vi "GeoData.vi"() -> ()   [LabVIEW 2017] (continued)
County\tH1\n26037\t54009\tFollansbee\tWV\tBrooke County\tH1\n26075\t54009\tWindsor heights\tWV\tBrooke County\tH1\n26062\t54009\tWeirton\tWV\tBrooke County\tH1\n26003\t54009\tWheeling\tWV\tBrooke County\tH1\n26030\t54009\tBeech bottom\tWV\tBrooke County\tH1\n26032\t54009\tBethany\tWV\tBrooke County\tH1\n26035\t54009\tColliers\tWV\tBrooke County\tH1\n26058\t54009\tShort creek\tWV\tBrooke County\tH1\n25504\t54011\tBarboursville\tWV\tCabell County\tH1\n25701\t54011\tHuntington\tWV\tCabell County\tH1\n25704\t54011\tHuntington\tWV\tCabell County\tH1\n26505\t54011\tMorgantown\tWV\tCabell County\tH1\n25723\t54011\tHuntington\tWV\tCabell County\tH1\n25711\t54011\tHuntington\tWV\tCabell County\tH1\n25727\t54011\tHuntington\tWV\tCabell County\tH1\n25702\t54011\tHuntington\tWV\tCabell County\tH1\n25703\t54011\tHuntington\tWV\tCabell County\tH1\n25713\t54011\tHuntington\tWV\tCabell County\tH1\n25779\t54011\tHuntington\tWV\tCabell County\tH1\n25772\t54011\tHuntington\tWV\tCabell County\tH1\n25716\t54011\tHuntington\tWV\tCabell County\tH1\n25715\t54011\tHuntington\tWV\tCabell County\tH1\n25526\t54011\tHurricane\tWV\tCabell County\tH1\n25510\t54011\tCulloden\tWV\tCabell County\tH1\n25714\t54011\tHuntington\tWV\tCabell County\tH1\n25778\t54011\tHuntington\tWV\tCabell County\tH1\n25728\t54011\tHuntington\tWV\tCabell County\tH1\n25755\t54011\tHuntington\tWV\tCabell County\tH1\n25706\t54011\tHuntington\tWV\tCabell County\tH1\n25719\t54011\tHuntington\tWV\tCabell County\tH1\n25729\t54011\tHuntington\tWV\tCabell County\tH1\n25775\t54011\tHuntington\tWV\tCabell County\tH1\n25545\t54011\tOna\tWV\tCabell County\tH1\n25708\t54011\tHuntington\tWV\tCabell County\tH1\n25721\t54011\tHuntington\tWV\tCabell County\tH1\n25726\t54011\tHuntington\tWV\tCabell County\tH1\n25725\t54011\tHuntington\tWV\tCabell County\tH1\n25717\t54011\tHuntington\tWV\tCabell County\tH1\n25773\t54011\tHuntington\tWV\tCabell County\tH1\n25541\t54011\tMilton\tWV\tCabell County\tH1\n25559\t54011\tSalt rock\tWV\tCabell County\tH1\n25520\t54011\tGlenwood\tWV\tCabell County\tH1\n25709\t54011\tHuntington\tWV\tCabell County\tH1\n25776\t54011\tHuntington\tWV\tCabell County\tH1\n25710\t54011\tHuntington\tWV\tCabell County\tH1\n25705\t54011\tHuntington\tWV\tCabell County\tH1\n25537\t54011\tLesage\tWV\tCabell County\tH1\n25777\t54011\tHuntington\tWV\tCabell County\tH1\n25707\t54011\tHuntington\tWV\tCabell County\tH1\n25712\t54011\tHuntington\tWV\tCabell County\tH1\n25722\t54011\tHuntington\tWV\tCabell County\tH1\n25506\t54011\tBranchland\tWV\tCabell County\tH1\n25718\t54011\tHuntington\tWV\tCabell County\tH1\n25720\t54011\tHuntington\tWV\tCabell County\tH1\n25724\t54011\tHuntington\tWV\tCabell County\tH1\n25774\t54011\tHuntington\tWV\tCabell County\tH1\n25235\t54013\tChloe\tWV\tCalhoun County\tH1\n25259\t54013\tLooneyville\tWV\tCalhoun County\tH1\n25261\t54013\tMillstone\tWV\tCalhoun County\tH1\n25141\t54013\tNebo\tWV\tCalhoun County\tH1\n26136\t54013\tBig bend\tWV\tCalhoun County\tH1\n25266\t54013\tNewton\tWV\tCalhoun County\tH1\n26147\t54013\tGrantsville\tWV\tCalhoun County\tH1\n26137\t54013\tBig springs\tWV\tCalhoun County\tH1\n26141\t54013\tCreston\tWV\tCalhoun County\tH1\n25234\t54013\tArnoldsburg\tWV\tCalhoun County\tH1\n26636\t54013\tRosedale\tWV\tCalhoun County\tH1\n26152\t54013\tMunday\tWV\tCalhoun County\tH1\n25276\t54013\tSpencer\tWV\tCalhoun County\tH1\n26151\t54013\tMount zion\tWV\tCalhoun County\tH1\n26138\t54013\tBrohard\tWV\tCalhoun County\tH1\n25268\t54013\tOrma\tWV\tCalhoun County\tH1\n25235\t54015\tChloe\tWV\tClay County\tH1\n25133\t54015\tMaysel\tWV\tClay County\tH1\n25125\t54015\tLizemores\tWV\tClay County\tH1\n25141\t54015\tNebo\tWV\tClay County\tH1\n25045\t54015\tClendenin\tWV\tClay County\tH1\n25043\t54015\tClay\tWV\tClay County\tH1\n25164\t54015\tProcious\tWV\tClay County\tH1\n25285\t54015\tWallback\tWV\tClay County\tH1\n25019\t54015\tBickmore\tWV\tClay County\tH1\n25088\t54015\tGlen\tWV\tClay County\tH1\n25113\t54015\tIvydale\tWV\tClay County\tH1\n25063\t54015\tDuck\tWV\tClay County\tH1\n26617\t54015\tDille\tWV\tClay County\tH1\n25111\t54015\tIndore\tWV\tClay County\tH1\n25030\t54015\tBomont\tWV\tClay County\tH1\n25211\t54015\tWiden\tWV\tClay County\tH1\n26321\t54017\tAlum bridge\tWV\tDoddridge County\tH1\n26443\t54017\tTroy\tWV\tDoddridge County\tH1\n26436\t54017\tSmithburg\tWV\tDoddridge County\tH1\n26415\t54017\tPennsboro\tWV\tDoddridge County\tH1\n26456\t54017\tWest union\tWV\tDoddridge County\tH1\n26411\t54017\tNew milton\tWV\tDoddridge County\tH1\n26426\t54017\tSalem\tWV\tDoddridge County\tH1\n26339\t54017\tCenter point\tWV\tDoddridge County\tH1\n26680\t54019\tNallen\tWV\tFayette County\tH1\n26656\t54019\tBelva\tWV\tFayette County\tH1\n25904\t54019\tPax\tWV\tFayette County\tH1\n25846\t54019\tGlen jean\tWV\tFayette County\tH1\n25002\t54019\tAlloy\tWV\tFayette County\tH1\n25031\t54019\tBoomer\tWV\tFayette County\tH1\n25801\t54019\tBeckley\tWV\tFayette County\tH1\n25840\t54019\tFayetteville\tWV\tFayette County\tH1\n25880\t54019\tMount hope\tWV\tFayette County\tH1\n26690\t54019\tSwiss\tWV\tFayette County\tH1\n25942\t54019\tWinona\tWV\tFayette County\tH1\n25936\t54019\tThurmond\tWV\tFayette County\tH1\n25901\t54019\tOak hill\tWV\tFayette County\tH1\n25119\t54019\tKincaid\tWV\tFayette County\tH1\n25186\t54019\tSmithers\tWV\tFayette County\tH1\n25831\t54019\tDanese\tWV\tFayette County\tH1\n25917\t54019\tScarbro\tWV\tFayette County\tH1\n25136\t54019\tMontgomery\tWV\tFayette County\tH1\n25083\t54019\tGallagher\tWV\tFayette County\tH1\n25115\t54019\tKanawha falls\tWV\tFayette County\tH1\n25938\t54019\tVictor\tWV\tFayette County\tH1\n25862\t54019\tLansing\tWV\tFayette County\tH1\n25139\t54019\tMount carbon\tWV\tFayette County\tH1\n25059\t54019\tDixie\tWV\tFayette County\tH1\n25866\t54019\tLochgelly\tWV\tFayette County\tH1\n25090\t54019\tGlen ferris\tWV\tFayette County\tH1\n25812\t54019\tAnsted\tWV\tFayette County\tH1\n25854\t54019\tHico\tWV\tFayette County\tH1\n25837\t54019\tEdmond\tWV\tFayette County\tH1\n25118\t54019\tKimberly\tWV\tFayette County\tH1\n25855\t54019\tHilltop\tWV\tFayette County\tH1\n25907\t54019\tPrince\tWV\tFayette County\tH1\n25879\t54019\tMinden\tWV\tFayette County\tH1\n25040\t54019\tCharlton heights\tWV\tFayette County\tH1\n25976\t54019\tMeadow bridge\tWV\tFayette County\tH1\n25161\t54019\tPowellton\tWV\tFayette County\tH1\n25173\t54019\tRobson\tWV\tFayette County\tH1\n25085\t54019\tGauley bridge\tWV\tFayette County\tH1\n25036\t54019\tCannelton\tWV\tFayette County\tH1\n25962\t54019\tRainelle\tWV\tFayette County\tH1\n25868\t54019\tLookout\tWV\tFayette County\tH1\n25185\t54019\tMount olive\tWV\tFayette County\tH1\n25888\t54019\tMount hope\tWV\tFayette County\tH1\n26412\t54021\tOrlando\tWV\tGilmer County\tH1\n26342\t54021\tCoxs mills\tWV\tGilmer County\tH1\n26384\t54021\tLinn\tWV\tGilmer County\tH1\n26443\t54021\tTroy\tWV\tGilmer County\tH1\n26638\t54021\tShock\tWV\tGilmer County\tH1\n26147\t54021\tGrantsville\tWV\tGilmer County\tH1\n26137\t54021\tBig springs\tWV\tGilmer County\tH1\n26335\t54021\tBurnsville\tWV\tGilmer County\tH1\n26430\t54021\tSand fork\tWV\tGilmer County\tH1\n26624\t54021\tGassaway\tWV\tGilmer County\tH1\n26611\t54021\tCedarville\tWV\tGilmer County\tH1\n26636\t54021\tRosedale\tWV\tGilmer County\tH1\n26351\t54021\tGlenville\tWV\tGilmer County\tH1\n26411\t54021\tNew milton\tWV\tGilmer County\tH1\n25267\t54021\tNormantown\tWV\tGilmer County\tH1\n26866\t54023\tUpper tract\tWV\tGrant County\tH1\n26717\t54023\tElk garden\tWV\tGrant County\tH1\n26855\t54023\tCabins\tWV\tGrant County\tH1\n26743\t54023\tNew creek\tWV\tGrant County\tH1\n26707\t54023\tBayard\tWV\tGrant County\tH1\n26739\t54023\tMount storm\tWV\tGrant County\tH1\n26720\t54023\tGormania\tWV\tGrant County\tH1\n26833\t54023\tMaysville\tWV\tGrant County\tH1\n26847\t54023\tPetersburg\tWV\tGrant County\tH1\n26836\t54023\tMoorefield\tWV\tGrant County\tH1\n26731\t54023\tLahmansville\tWV\tGrant County\tH1\n26710\t54023\tBurlington\tWV\tGrant County\tH1\n24977\t54025\tSmoot\tWV\tGreenbrier County\tH1\n26680\t54025\tNallen\tWV\tGreenbrier County\tH1\n24938\t54025\tFrankford\tWV\tGreenbrier County\tH1\n24901\t54025\tLewisburg\tWV\tGreenbrier County\tH1\n24931\t54025\tCrawley\tWV\tGreenbrier County\tH1\n26261\t54025\tRichwood\tWV\tGreenbrier County\tH1\n25981\t54025\tQuinwood\tWV\tGreenbrier County\tH1\n25984\t54025\tRupert\tWV\tGreenbrier County\tH1\n24966\t54025\tRenick\tWV\tGreenbrier County\tH1\n24957\t54025\tMaxwelton\tWV\tGreenbrier County\tH1\n24954\t54025\tMarlinton\tWV\tGreenbrier County\tH1\n24925\t54025\tCaldwell\tWV\tGreenbrier County\tH1\n24970\t54025\tRonceverte\tWV\tGreenbrier County\tH1\n25958\t54025\tCharmco\tWV\tGreenbrier County\tH1\n24916\t54025\tAsbury\tWV\tGreenbrier County\tH1\n25976\t54025\tMeadow bridge\tWV\tGreenbrier County\tH1\n24910\t54025\tAlderson\tWV\tGreenbrier County\tH1\n24986\t54025\tWhite sulphur springs\tWV\tGreenbrier County\tH1\n25962\t54025\tRainelle\tWV\tGreenbrier County\tH1\n24991\t54025\tWilliamsburg\tWV\tGreenbrier County\tH1\n24943\t54025\tGrassy meadows\tWV\tGreenbrier County\tH1\n25972\t54025\tLeslie\tWV\tGreenbrier County\tH1\n25434\t54027\tPaw paw\tWV\tHampshire County\tH1\n25422\t54027\tGreat cacapon\tWV\tHampshire County\tH1\n26704\t54027\tAugusta\tWV\tHampshire County\tH1\n26755\t54027\tRio\tWV\tHampshire County\tH1\n26711\t54027\tCapon bridge\tWV\tHampshire County\tH1\n26761\t54027\tShanks\tWV\tHampshire County\tH1\n26852\t54027\tPurgitsville\tWV\tHampshire County\tH1\n25437\t54027\tPoints\tWV\tHampshire County\tH1\n25431\t54027\tLevels\tWV\tHampshire County\tH1\n26808\t54027\tHigh view\tWV\tHampshire County\tH1\n26722\t54027\tGreen spring\tWV\tHampshire County\tH1\n26763\t54027\tSpringfield\tWV\tHampshire County\tH1\n26823\t54027\tCapon springs\tWV\tHampshire County\tH1\n25444\t54027\tSlanesville\tWV\tHampshire County\tH1\n26865\t54027\tYellow spring\tWV\tHampshire County\tH1\n26817\t54027\tBloomery\tWV\tHampshire County\tH1\n26757\t54027\tRomney\tWV\tHampshire County\tH1\n26710\t54027\tBurlington\tWV\tHampshire County\tH1\n26714\t54027\tDelray\tWV\tHampshire County\tH1\n26047\t54029\tNew cumberland\tWV\tHancock County\tH1\n26062\t54029\tWeirton\tWV\tHancock County\tH1\n26050\t54029\tNewell\tWV\tHancock County\tH1\n26056\t54029\tNew manchester\tWV\tHancock County\tH1\n26034\t54029\tChester\tWV\tHancock County\tH1\n26838\t54031\tMilam\tWV\tHardy County\tH1\n26755\t54031\tRio\tWV\tHardy County\tH1\n26851\t54031\tWardensville\tWV\tHardy County\tH1\n26818\t54031\tFisher\tWV\tHardy County\tH1\n26852\t54031\tPurgitsville\tWV\tHardy County\tH1\n26810\t54031\tLost city\tWV\tHardy County\tH1\n26845\t54031\tOld fields\tWV\tHardy County\tH1\n26812\t54031\tMathias\tWV\tHardy County\tH1\n26801\t54031\tBaker\tWV\tHardy County\tH1\n26847\t54031\tPetersburg\tWV\tHardy County\tH1\n26836\t54031\tMoorefield\tWV\tHardy County\tH1\n26815\t54031\tSugar grove\tWV\tHardy County\tH1\n26323\t54033\tAnmoore\tWV\tHarrison County\tH1\n26301\t54033\tClarksburg\tWV\tHarrison County\tH1\n26330\t54033\tBridgeport\tWV\tHarrison County\tH1\n26385\t54033\tLost creek\tWV\tHarrison County\tH1\n26416\t54033\tPhilippi\tWV\tHarrison County\tH1\n26361\t54033\tGypsy\tWV\tHarrison County\tH1\n26378\t54033\tJane lew\tWV\tHarrison County\tH1\n26582\t54033\tMannington\tWV\tHarrison County\tH1\n26386\t54033\tLumberport\tWV\tHarrison County\tH1\n26451\t54033\tWest milford\tWV\tHarrison County\tH1\n26456\t54033\tWest union\tWV\tHarrison County\tH1\n26438\t54033\tSpelter\tWV\tHarrison County\tH1\n26591\t54033\tWorthington\tWV\tHarrison County\tH1\n26422\t54033\tReynoldsville\tWV\tHarrison County\tH1\n26554\t54033\tFairmont\tWV\tHarrison County\tH1\n26568\t54033\tEnterprise\tWV\tHarrison County\tH1\n26306\t54033\tClarksburg\tWV\tHarrison County\tH1\n26426\t54033\tSalem\tWV\tHarrison County\tH1\n26366\t54033\tHaywood\tWV\tHarrison County\tH1\n26369\t54033\tHepzibah\tWV\tHarrison County\tH1\n26463\t54033\tWyatt\tWV\tHarrison County\tH1\n26408\t54033\tMount clare\tWV\tHarrison County\tH1\n26431\t54033\tShinnston\tWV\tHarrison County\tH1\n26448\t54033\tWallace\tWV\tHarrison County\tH1\n26404\t54033\tMeadowbrook\tWV\tHarrison County\tH1\n25252\t54035\tLe roy\tWV\tJackson County\tH1\n26169\t54035\tRockport\tWV\tJackson County\tH1\n25271\t54035\tRipley\tWV\tJackson County\tH1\n26164\t54035\tRavenswood\tWV\tJackson County\tH1\n25275\t54035\tSandyville\tWV\tJackson County\tH1\n25264\t54035\tMount alto\tWV\tJackson County\tH1\n25262\t54035\tMillwood\tWV\tJackson County\tH1\n25244\t54035\tGay\tWV\tJackson County\tH1\n25243\t54035\tGandeeville\tWV\tJackson County\tH1\n26143\t54035\tElizabeth\tWV\tJackson County\tH1\n26160\t54035\tPalestine\tWV\tJackson County\tH1\n25245\t54035\tGiven\tWV\tJackson County\tH1\n25241\t54035\tEvans\tWV\tJackson County\tH1\n25248\t54035\tKenna\tWV\tJackson County\tH1\n25124\t54035\tLiberty\tWV\tJackson County\tH1\n26133\t54035\tBelleville\tWV\tJackson County\tH1\n25239\t54035\tCottageville\tWV\tJackson County\tH1\n25231\t54035\tAdvent\tWV\tJackson County\tH1\n25414\t54037\tCharles town\tWV\tJefferson County\tH1\n25425\t54037\tHarpers ferry\tWV\tJefferson County\tH1\n25446\t54037\tSummit point\tWV\tJefferson County\tH1\n25443\t54037\tShepherdstown\tWV\tJefferson County\tH1\n25441\t54037\tRippon\tWV\tJefferson County\tH1\n25404\t54037\tMartinsburg\tWV\tJefferson County\tH1\n25442\t54037\tShenandoah junction\tWV\tJefferson County\tH1\n25432\t54037\tMillville\tWV\tJefferson County\tH1\n25430\t54037\tKearneysville\tWV\tJefferson County\tH1\n25438\t54037\tRanson\tWV\tJefferson County\tH1\n25423\t54037\tHalltown\tWV\tJefferson County\tH1\n25071\t54039\tElkview\tWV\tKanawha County\tH1\n25301\t54039\tCharleston\tWV\tKanawha County\tH1\n25312\t54039\tCharleston\tWV\tKanawha County\tH1\n25311\t54039\tCharleston\tWV\tKanawha County\tH1\n25320\t54039\tCharleston\tWV\tKanawha County\tH1\n25324\t54039\tCharleston\tWV\tKanawha County\tH1\n25326\t54039\tCharleston\tWV\tKanawha County\tH1\n25334\t54039\tCharleston\tWV\tKanawha County\tH1\n25336\t54039\tCharleston\tWV\tKanawha County\tH1\n25102\t54039\tHandley\tWV\tKanawha County\tH1\n25201\t54039\tTad\tWV\tKanawha County\tH1\n25143\t54039\tNitro\tWV\tKanawha County\tH1\n25075\t54039\tEskdale\tWV\tKanawha County\tH1\n25213\t54039\tWinfield\tWV\tKanawha County\tH1\n25303\t54039\tSouth charleston\tWV\tKanawha County\tH1\n25339\t54039\tCharleston\tWV\tKanawha County\tH1\n25321\t54039\tCharleston\tWV\tKanawha County\tH1\n25112\t54039\tInstitute\tWV\tKanawha County\tH1\n25327\t54039\tCharleston\tWV\tKanawha County\tH1\n25322\t54039\tCharleston\tWV\tKanawha County\tH1\n25328\t54039\tCharleston\tWV\tKanawha County\tH1\n25126\t54039\tLondon\tWV\tKanawha County\tH1\n25314\t54039\tCharleston\tWV\tKanawha County\tH1\n25306\t54039\tCharleston\tWV\tKanawha County\tH1\n25039\t54039\tCedar grove\tWV\tKanawha County\tH1\n25364\t54039\tCharleston\tWV\tKanawha County\tH1\n25361\t54039\tCharleston\tWV\tKanawha County\tH1\n25323\t54039\tCharleston\tWV\tKanawha County\tH1\n25335\t54039\tCharleston\tWV\tKanawha County\tH1\n25338\t54039\tCharleston\tWV\tKanawha County\tH1\n25045\t54039\tClendenin\tWV\tKanawha County\tH1\n25202\t54039\tTornado\tWV\tKanawha County\tH1\n25309\t54039\tSouth charleston\tWV\tKanawha County\tH1\n25286\t54039\tWalton\tWV\tKanawha County\tH1\n25387\t54039\tCharleston\tWV\tKanawha County\tH1\n25162\t54039\tPratt\tWV\tKanawha County\tH1\n25333\t54039\tCharleston\tWV\tKanawha County\tH1\n25362\t54039\tCharleston\tWV\tKanawha County\tH1\n25136\t54039\tMontgomery\tWV\tKanawha County\tH1\n25110\t54039\tHugheston\tWV\tKanawha County\tH1\n25083\t54039\tGallagher\tWV\tKanawha County\tH1\n25054\t54039\tDawes\tWV\tKanawha County\tH1\n25331\t54039\tCharleston\tWV\tKanawha County\tH1\n25159\t54039\tPoca\tWV\tKanawha County\tH1\n25305\t54039\tCharleston\tWV\tKanawha County\tH1\n25313\t54039\tCharleston\tWV\tKanawha County\tH1\n25330\t54039\tCharleston\tWV\tKanawha County\tH1\n25332\t54039\tCharleston\tWV\tKanawha County\tH1\n25325\t54039\tCharleston\tWV\tKanawha County\tH1\n25026\t54039\tBlue creek\tWV\tKanawha County\tH1\n25302\t54039\tCharleston\tWV\tKanawha County\tH1\n25025\t54039\tBlount\tWV\tKanawha County\tH1\n25160\t54039\tPond gap\tWV\tKanawha County\tH1\n25337\t54039\tCharleston\tWV\tKanawha County\tH1\n25317\t54039\tCharleston\tWV\tKanawha County\tH1\n25064\t54039\tDunbar\tWV\tKanawha County\tH1\n25177\t54039\tSaint albans\tWV\tKanawha County\tH1\n25248\t54039\tKenna\tWV\tKanawha County\tH1\n25124\t54039\tLiberty\tWV\tKanawha County\tH1\n25304\t54039\tCharleston\tWV\tKanawha County\tH1\n25107\t54039\tHernshaw\tWV\tKanawha County\tH1\n25389\t54039\tCharleston\tWV\tKanawha County\tH1\n25035\t54039\tCabin creek\tWV\tKanawha County\tH1\n25067\t54039\tEast bank\tWV\tKanawha County\tH1\n25061\t54039\tDrybranch\tWV\tKanawha County\tH1\n25015\t54039\tBelle\tWV\tKanawha County\tH1\n25003\t54039\tAlum creek\tWV\tKanawha County\tH1\n25214\t54039\tWinifrede\tWV\tKanawha County\tH1\n25315\t54039\tCharleston\tWV\tKanawha County\tH1\n25030\t54039\tBomont\tWV\tKanawha County\tH1\n25132\t54039\tMammoth\tWV\tKanawha County\tH1\n25103\t54039\tHansford\tWV\tKanawha County\tH1\n25329\t54039\tCharleston\tWV\tKanawha County\tH1\n25156\t54039\tPinch\tWV\tKanawha County\tH1\n25079\t54039\tFalling rock\tWV\tKanawha County\tH1\n25086\t54039\tGlasgow\tWV\tKanawha County\tH1\n25134\t54039\tMiami\tWV\tKanawha County\tH1\n25396\t54039\tCharleston\tWV\tKanawha County\tH1\n26321\t54041\tAlum bridge\tWV\tLewis County\tH1\n26412\t54041\tOrlando\tWV\tLewis County\tH1\n26384\t54041\tLinn\tWV\tLewis County\tH1\n26218\t54041\tFrench creek\tWV\tLewis County\tH1\n26372\t54041\tHorner\tWV\tLewis County\tH1\n26376\t54041\tIreland\tWV\tLewis County\tH1\n26378\t54041\tJane lew\tWV\tLewis County\tH1\n26452\t54041\tWeston\tWV\tLewis County\tH1\n26338\t54041\tCamden\tWV\tLewis County\tH1\n26447\t54041\tWalkersville\tWV\tLewis County\tH1\n26201\t54041\tBuckhannon\tWV\tLewis County\tH1\n26343\t54041\tCrawford\tWV\tLewis County\tH1\n26411\t54041\tNew milton\tWV\tLewis County\tH1\n25523\t54043\tHamlin\tWV\tLincoln County\tH1\n25529\t54043\tJulian\tWV\tLincoln County\tH1\n25521\t54043\tGriffithsville\tWV\tLincoln County\tH1\n25564\t54043\tSod\tWV\tLincoln County\tH1\n25526\t54043\tHurricane\tWV\tLincoln County\tH1\n25510\t54043\tCulloden\tWV\tLincoln County\tH1\n25573\t54043\tYawkey\tWV\tLincoln County\tH1\n25699\t54043\tWilsondale\tWV\tLincoln County\tH1\n25202\t54043\tTornado\tWV\tLincoln County\tH1\n25501\t54043\tAlkol\tWV\tLincoln County\tH1\n25524\t54043\tHarts\tWV\tLincoln County\tH1\n25313\t54043\tCharleston\tWV\tLincoln County\tH1\n25565\t54043\tSpurlockville\tWV\tLincoln County\tH1\n25567\t54043\tSumerco\tWV\tLincoln County\tH1\n25534\t54043\tKiahsville\tWV\tLincoln County\tH1\n25557\t54043\tRanger\tWV\tLincoln County\tH1\n25571\t54043\tWest hamlin\tWV\tLincoln County\tH1\n25540\t54043\tMidkiff\tWV\tLincoln County\tH1\n25544\t54043\tMyra\tWV\tLincoln County\tH1\n25003\t54043\tAlum creek\tWV\tLincoln County\tH1\n25506\t54043\tBranchland\tWV\tLincoln County\tH1\n25617\t54045\tDavin\tWV\tLogan County\tH1\n25634\t54045\tMallory\tWV\tLogan County\tH1\n25625\t54045\tHolden\tWV\tLogan County\tH1\n25505\t54045\tBig creek\tWV\tLogan County\tH1\n25612\t54045\tChauncey\tWV\tLogan County\tH1\n25653\t54045\tWilkinson\tWV\tLogan County\tH1\n25508\t54045\tChapmanville\tWV\tLogan County\tH1\n25547\t54045\tPecks mill\tWV\tLogan County\tH1\n25644\t54045\tSarah ann\tWV\tLogan County\tH1\n25022\t54045\tBlair\tWV\tLogan County\tH1\n25628\t54045\tKistler\tWV\tLogan County\tH1\n25524\t54045\tHarts\tWV\tLogan County\tH1\n25646\t54045\tStollings\tWV\tLogan County\tH1\n25047\t54045\tClothier\tWV\tLogan County\tH1\n25647\t54045\tSwitzer\tWV\tLogan County\tH1\n25639\t54045\tPeach creek\tWV\tLogan County\tH1\n25108\t54045\tHewett\tWV\tLogan County\tH1\n25652\t54045\tWhitman\tWV\tLogan County\tH1\n25606\t54045\tAccoville\tWV\tLogan County\tH1\n25614\t54045\tCora\tWV\tLogan County\tH1\n25649\t54045\tVerdunville\tWV\tLogan County\tH1\n25654\t54045\tYolyn\tWV\tLogan County\tH1\n25635\t54045\tMan\tWV\tLogan County\tH1\n25183\t54045\tSharples\tWV\tLogan County\tH1\n25607\t54045\tAmherstdale\tWV\tLogan County\tH1\n25601\t54045\tLogan\tWV\tLogan County\tH1\n25638\t54045\tOmar\tWV\tLogan County\tH1\n25121\t54045\tLake\tWV\tLogan County\tH1\n25670\t54045\tDelbarton\tWV\tLogan County\tH1\n25076\t54045\tEthel\tWV\tLogan County\tH1\n25632\t54045\tLyburn\tWV\tLogan County\tH1\n25637\t54045\tMount gay\tWV\tLogan County\tH1\n25611\t54045\tBruno\tWV\tLogan County\tH1\n25624\t54045\tHenlawson\tWV\tLogan County\tH1\n25630\t54045\tLorado\tWV\tLogan County\tH1\n24862\t54047\tMohawk\tWV\tMcDowell County\tH1\n24871\t54047\tPageton\tWV\tMcDowell County\tH1\n24831\t54047\tElkhorn\tWV\tMcDowell County\tH1\n24861\t54047\tMaybeury\tWV\tMcDowell County\tH1\n24881\t54047\tRoderfield\tWV\tMcDowell County\tH1\n24866\t54047\tNewhall\tWV\tMcDowell County\tH1\n24813\t54047\tBartley\tWV\tMcDowell County\tH1\n24811\t54047\tAvondale\tWV\tMcDowell County\tH1\n24817\t54047\tBradshaw\tWV\tMcDowell County\tH1\n24826\t54047\tCucumber\tWV\tMcDowell County\tH1\n24828\t54047\tDavy\tWV\tMcDowell County\tH1\n24879\t54047\tRaysal\tWV\tMcDowell County\tH1\n24846\t54047\tIsaban\tWV\tMcDowell County\tH1\n24855\t54047\tKyle\tWV\tMcDowell County\tH1\n24830\t54047\tElbert\tWV\tMcDowell County\tH1\n24829\t54047\tEckman\tWV\tMcDowell County\tH1\n24816\t54047\tBig sandy\tWV\tMcDowell County\tH1\n24873\t54047\tPaynesville\tWV\tMcDowell County\tH1\n24895\t54047\tWilcoe\tWV\tMcDowell County\tH1\n24878\t54047\tPremier\tWV\tMcDowell County\tH1\n24894\t54047\tWarriormine\tWV\tMcDowell County\tH1\n24808\t54047\tAnawalt\tWV\tMcDowell County\tH1\n24848\t54047\tJenkinjones\tWV\tMcDowell County\tH1\n24836\t54047\tGary\tWV\tMcDowell County\tH1\n24892\t54047\tWar\tWV\tMcDowell County\tH1\n24801\t54047\tWelch\tWV\tMcDowell County\tH1\n24872\t54047\tPanther\tWV\tMcDowell County\tH1\n24868\t54047\tNorthfork\tWV\tMcDowell County\tH1\n24815\t54047\tBerwind\tWV\tMcDowell County\tH1\n24850\t54047\tJolo\tWV\tMcDowell County\tH1\n24888\t54047\tThorpe\tWV\tMcDowell County\tH1\n24884\t54047\tSquire\tWV\tMcDowell County\tH1\n24844\t54047\tIaeger\tWV\tMcDowell County\tH1\n24853\t54047\tKimball\tWV\tMcDowell County\tH1\n24843\t54047\tHensley\tWV\tMcDowell County\tH1\n24887\t54047\tSwitchback\tWV\tMcDowell County\tH1\n26563\t54049\tCarolina\tWV\tMarion County\tH1\n26330\t54049\tBridgeport\tWV\tMarion County\tH1\n26508\t54049\tMorgantown\tWV\tMarion County\tH1\n26570\t54049\tFairview\tWV\tMarion County\tH1\n26588\t54049\tRivesville\tWV\tMarion County\tH1\n26562\t54049\tBurton\tWV\tMarion County\tH1\n26586\t54049\tMontana mines\tWV\tMarion County\tH1\n26559\t54049\tBarrackville\tWV\tMarion County\tH1\n26354\t54049\tGrafton\tWV\tMarion County\tH1\n26582\t54049\tMannington\tWV\tMarion County\tH1\n26576\t54049\tIdamay\tWV\tMarion County\tH1\n26572\t54049\tFour states\tWV\tMarion County\tH1\n26555\t54049\tFairmont\tWV\tMarion County\tH1\n26585\t54049\tMetz\tWV\tMarion County\tH1\n26571\t54049\tFarmington\tWV\tMarion County\tH1\n26591\t54049\tWorthington\tWV\tMarion County\tH1\n26561\t54049\tBig run\tWV\tMarion County\tH1\n26578\t54049\tKingmont\tWV\tMarion County\tH1\n26554\t54049\tFairmont\tWV\tMarion County\tH1\n26574\t54049\tGrant town\tWV\tMarion County\tH1\n26566\t54049\tColfax\tWV\tMarion County\tH1\n26587\t54049\tRachel\tWV\tMarion County\tH1\n26448\t54049\tWallace\tWV\tMarion County\tH1\n26560\t54049\tBaxter\tWV\tMarion County\tH1\n26036\t54051\tDallas\tWV\tMarshall County\tH1\n26033\t54051\tCameron\tWV\tMarshall County\tH1\n26003\t54051\tWheeling\tWV\tMarshall County\tH1\n26040\t54051\tMcmechen\tWV\tMarshall County\tH1\n26041\t54051\tMoundsville\tWV\tMarshall County\tH1\n26055\t54051\tProctor\tWV\tMarshall County\tH1\n26039\t54051\tGlen easton\tWV\tMarshall County\tH1\n26031\t54051\tBenwood\tWV\tMarshall County\tH1\n26038\t54051\tGlen dale\tWV\tMarshall County\tH1\n25515\t54053\tGallipolis ferry\tWV\tMason County\tH1\n25106\t54053\tHenderson\tWV\tMason County\tH1\n25265\t54053\tNew haven\tWV\tMason County\tH1\n25264\t54053\tMount alto\tWV\tMason County\tH1\n25502\t54053\tApple grove\tWV\tMason County\tH1\n25503\t54053\tAshton\tWV\tMason County\tH1\n25253\t54053\tLetart\tWV\tMason County\tH1\n25123\t54053\tLeon\tWV\tMason County\tH1\n25541\t54053\tMilton\tWV\tMason County\tH1\n25520\t54053\tGlenwood\tWV\tMason County\tH1\n25247\t54053\tHartford\tWV\tMason County\tH1\n25082\t54053\tFraziers bottom\tWV\tMason County\tH1\n25187\t54053\tSouthside\tWV\tMason County\tH1\n25241\t54053\tEvans\tWV\tMason County\tH1\n25260\t54053\tMason\tWV\tMason County\tH1\n25287\t54053\tWest columbia\tWV\tMason County\tH1\n25550\t54053\tPoint pleasant\tWV\tMason County\tH1\n25239\t54053\tCottageville\tWV\tMason County\tH1\n24701\t54055\tBluefield\tWV\tMercer County\tH1\n25922\t54055\tSpanishburg\tWV\tMercer County\tH1\n24712\t54055\tAthens\tWV\tMercer County\tH1\n24732\t54055\tKellysville\tWV\tMercer County\tH1\n24729\t54055\tHiawatha\tWV\tMercer County\tH1\n24738\t54055\tNemours\tWV\tMercer County\tH1\n24739\t54055\tPrinceton\tWV\tMercer County\tH1\n25971\t54055\tLerona\tWV\tMercer County\tH1\n25979\t54055\tPipestem\tWV\tMercer County\tH1\n24737\t54055\tMontcalm\tWV\tMercer County\tH1\n25841\t54055\tFlat top\tWV\tMercer County\tH1\n24733\t54055\tLashmeet\tWV\tMercer County\tH1\n24715\t54055\tBramwell\tWV\tMercer County\tH1\n24740\t54055\tPrinceton\tWV\tMercer County\tH1\n24747\t54055\tRock\tWV\tMercer County\tH1\n24736\t54055\tMatoaka\tWV\tMercer County\tH1\n25820\t54055\tCamp creek\tWV\tMercer County\tH1\n24714\t54055\tBeeson\tWV\tMercer County\tH1\n24731\t54055\tKegley\tWV\tMercer County\tH1\n25902\t54055\tOdd\tWV\tMercer County\tH1\n24724\t54055\tFreeman\tWV\tMercer County\tH1\n26767\t54057\tWiley ford\tWV\tMineral County\tH1\n26726\t54057\tKeyser\tWV\tMineral County\tH1\n26717\t54057\tElk garden\tWV\tMineral County\tH1\n26750\t54057\tPiedmont\tWV\tMineral County\tH1\n26852\t54057\tPurgitsville\tWV\tMineral County\tH1\n26753\t54057\tRidgeley\tWV\tMineral County\tH1\n26763\t54057\tSpringfield\tWV\tMineral County\tH1\n26743\t54057\tNew creek\tWV\tMineral County\tH1\n26757\t54057\tRomney\tWV\tMineral County\tH1\n26719\t54057\tFort ashby\tWV\tMineral County\tH1\n26731\t54057\tLahmansville\tWV\tMineral County\tH1\n26710\t54057\tBurlington\tWV\tMineral County\tH1\n25678\t54059\tMatewan\tWV\tMingo County\tH1\n25672\t54059\tEdgarton\tWV\tMingo County\tH1\n25651\t54059\tWharncliffe\tWV\tMingo County\tH1\n25685\t54059\tNaugatuck\tWV\tMingo County\tH1\n25667\t54059\tChattaroy\tWV\tMingo County\tH1\n25691\t54059\tRawl\tWV\tMingo County\tH1\n25676\t54059\tLenore\tWV\tMingo County\tH1\n25686\t54059\tNewtown\tWV\tMingo County\tH1\n25661\t54059\tWilliamson\tWV\tMingo County\tH1\n25666\t54059\tBreeden\tWV\tMingo County\tH1\n24851\t54059\tJustice\tWV\tMingo County\tH1\n25671\t54059\tDingess\tWV\tMingo County\tH1\n25688\t54059\tNorth matewan\tWV\tMingo County\tH1\n25650\t54059\tVerner\tWV\tMingo County\tH1\n25692\t54059\tRed jacket\tWV\tMingo County\tH1\n25608\t54059\tBaisden\tWV\tMingo County\tH1\n25696\t54059\tVarney\tWV\tMingo County\tH1\n25690\t54059\tRagland\tWV\tMingo County\tH1\n25670\t54059\tDelbarton\tWV\tMingo County\tH1\n25674\t54059\tKermit\tWV\tMingo County\tH1\n25621\t54059\tGilbert\tWV\tMingo County\tH1\n26505\t54061\tMorgantown\tWV\tMonongalia County\tH1\n26542\t54061\tMasontown\tWV\tMonongalia County\tH1\n26506\t54061\tMorgantown\tWV\tMonongalia County\tH1\n26374\t54061\tIndependence\tWV\tMonongalia County\tH1\n26508\t54061\tMorgantown\tWV\tMonongalia County\tH1\n26570\t54061\tFairview\tWV\tMonongalia County\tH1\n26588\t54061\tRivesville\tWV\tMonongalia County\tH1\n26562\t54061\tBurton\tWV\tMonongalia County\tH1\n26544\t54061\tPentress\tWV\tMonongalia County\tH1\n26354\t54061\tGrafton\tWV\tMonongalia County\tH1\n26582\t54061\tMannington\tWV\tMonongalia County\tH1\n26531\t54061\tDellslow\tWV\tMonongalia County\tH1\n26501\t54061\tMorgantown\tWV\tMonongalia County\tH1\n26585\t54061\tMetz\tWV\tMonongalia County\tH1\n26546\t54061\tPursglove\tWV\tMonongalia County\tH1\n26554\t54061\tFairmont\tWV\tMonongalia County\tH1\n26525\t54061\tBruceton mills\tWV\tMonongalia County\tH1\n26590\t54061\tWana\tWV\tMonongalia County\tH1\n26543\t54061\tOsage\tWV\tMonongalia County\tH1\n26534\t54061\tGranville\tWV\tMonongalia County\tH1\n26541\t54061\tMaidsville\tWV\tMonongalia County\tH1\n26507\t54061\tMorgantown\tWV\tMonongalia County\tH1\n26504\t54061\tMorgantown\tWV\tMonongalia County\tH1\n26521\t54061\tBlacksville\tWV\tMonongalia County\tH1\n26527\t54061\tCassville\tWV\tMonongalia County\tH1\n24963\t54063\tPeterstown\tWV\tMonroe County\tH1\n24984\t54063\tWaiteville\tWV\tMonroe County\tH1\n24918\t54063\tBallard\tWV\tMonroe County\tH1\n24945\t54063\tGreenville\tWV\tMonroe County\tH1\n24983\t54063\tUnion\tWV\tMonroe County\tH1\n24976\t54063\tSinks grove\tWV\tMonroe County\tH1\n24951\t54063\tLindside\tWV\tMonroe County\tH1\n24941\t54063\tGap mills\tWV\tMonroe County\tH1\n24985\t54063\tWayside\tWV\tMonroe County\tH1\n24974\t54063\tSecondcreek\tWV\tMonroe County\tH1\n24910\t54063\tAlderson\tWV\tMonroe County\tH1\n24993\t54063\tWolfcreek\tWV\tMonroe County\tH1\n25411\t54065\tBerkeley springs\tWV\tMorgan County\tH1\n25434\t54065\tPaw paw\tWV\tMorgan County\tH1\n25422\t54065\tGreat cacapon\tWV\tMorgan County\tH1\n25427\t54065\tHedgesville\tWV\tMorgan County\tH1\n26205\t54067\tCraigsville\tWV\tNicholas County\tH1\n26601\t54067\tSutton\tWV\tNicholas County\tH1\n26651\t54067\tSummersville\tWV\tNicholas County\tH1\n26681\t54067\tNettie\tWV\tNicholas County\tH1\n26680\t54067\tNallen\tWV\tNicholas County\tH1\n26656\t54067\tBelva\tWV\tNicholas County\tH1\n26202\t54067\tFenwick\tWV\tNicholas County\tH1\n26660\t54067\tCalvin\tWV\tNicholas County\tH1\n26690\t54067\tSwiss\tWV\tNicholas County\tH1\n26261\t54067\tRichwood\tWV\tNicholas County\tH1\n26676\t54067\tLeivasy\tWV\tNicholas County\tH1\n26691\t54067\tTioga\tWV\tNicholas County\tH1\n25981\t54067\tQuinwood\tWV\tNicholas County\tH1\n26667\t54067\tDrennen\tWV\tNicholas County\tH1\n25043\t54067\tClay\tWV\tNicholas County\tH1\n26208\t54067\tCamden on gauley\tWV\tNicholas County\tH1\n26678\t54067\tMount lookout\tWV\tNicholas County\tH1\n26610\t54067\tBirch river\tWV\tNicholas County\tH1\n26675\t54067\tKeslers cross lanes\tWV\tNicholas County\tH1\n26684\t54067\tPool\tWV\tNicholas County\tH1\n25059\t54067\tDixie\tWV\tNicholas County\tH1\n26671\t54067\tGilboa\tWV\tNicholas County\tH1\n26662\t54067\tCanvas\tWV\tNicholas County\tH1\n25063\t54067\tDuck\tWV\tNicholas County\tH1\n26679\t54067\tMount nebo\tWV\tNicholas County\tH1\n26070\t54069\tWellsburg\tWV\tOhio County\tH1\n26059\t54069\tTriadelphia\tWV\tOhio County\tH1\n26003\t54069\tWheeling\tWV\tOhio County\tH1\n26032\t54069\tBethany\tWV\tOhio County\tH1\n26074\t54069\tWest liberty\tWV\tOhio County\tH1\n26041\t54069\tMoundsville\tWV\tOhio County\tH1\n26060\t54069\tValley grove\tWV\tOhio County\tH1\n26031\t54069\tBenwood\tWV\tOhio County\tH1\n25003\t54069\tAlum creek\tWV\tOhio County\tH1\n26807\t54071\tFranklin\tWV\tPendleton County\tH1\n26866\t54071\tUpper tract\tWV\tPendleton County\tH1\n26804\t54071\tCircleville\tWV\tPendleton County\tH1\n26886\t54071\tOnego\tWV\tPendleton County\tH1\n26884\t54071\tSeneca rocks\tWV\tPendleton County\tH1\n26847\t54071\tPetersburg\tWV\tPendleton County\tH1\n26815\t54071\tSugar grove\tWV\tPendleton County\tH1\n26814\t54071\tRiverton\tWV\tPendleton County\tH1\n26802\t54071\tBrandywine\tWV\tPendleton County\tH1\n26170\t54073\tSaint marys\tWV\tPleasants County\tH1\n26184\t54073\tWaverly\tWV\tPleasants County\tH1\n26346\t54073\tEllenboro\tWV\tPleasants County\tH1\n26134\t54073\tBelmont\tWV\tPleasants County\tH1\n26146\t54073\tFriendly\tWV\tPleasants County\tH1\n24924\t54075\tBuckeye\tWV\tPocahontas County\tH1\n26294\t54075\tValley head\tWV\tPocahontas County\tH1\n24944\t54075\tGreen bank\tWV\tPocahontas County\tH1\n26253\t54075\tBeverly\tWV\tPocahontas County\tH1\n26273\t54075\tHuttonsville\tWV\tPocahontas County\tH1\n24915\t54075\tArbovale\tWV\tPocahontas County\tH1\n24927\t54075\tCass\tWV\tPocahontas County\tH1\n24946\t54075\tHillsboro\tWV\tPocahontas County\tH1\n24954\t54075\tMarlinton\tWV\tPocahontas County\tH1\n26282\t54075\tMonterville\tWV\tPocahontas County\tH1\n24934\t54075\tDunmore\tWV\tPocahontas County\tH1\n26264\t54075\tDurbin\tWV\tPocahontas County\tH1\n24986\t54075\tWhite sulphur springs\tWV\tPocahontas County\tH1\n24920\t54075\tBartow\tWV\tPocahontas County\tH1\n26291\t54075\tSlatyfork\tWV\tPocahontas County\tH1\n26287\t54077\tParsons\tWV\tPreston County\tH1\n26425\t54077\tRowlesburg\tWV\tPreston County\tH1\n26519\t54077\tAlbright\tWV\tPreston County\tH1\n26542\t54077\tMasontown\tWV\tPreston County\tH1\n26764\t54077\tTerra alta\tWV\tPreston County\tH1\n26716\t54077\tEglon\tWV\tPreston County\tH1\n26374\t54077\tIndependence\tWV\tPreston County\tH1\n26537\t54077\tKingwood\tWV\tPreston County\tH1\n26524\t54077\tBretz\tWV\tPreston County\tH1\n26547\t54077\tReedsville\tWV\tPreston County\tH1\n26410\t54077\tNewburg\tWV\tPreston County\tH1\n26405\t54077\tMoatsville\tWV\tPreston County\tH1\n26525\t54077\tBruceton mills\tWV\tPreston County\tH1\n26444\t54077\tTunnelton\tWV\tPreston County\tH1\n26440\t54077\tThornton\tWV\tPreston County\tH1\n26520\t54077\tArthurdale\tWV\tPreston County\tH1\n26705\t54077\tAurora\tWV\tPreston County\tH1\n25312\t54079\tCharleston\tWV\tPutnam County\tH1\n25523\t54079\tHamlin\tWV\tPutnam County\tH1\n25143\t54079\tNitro\tWV\tPutnam County\tH1\n25213\t54079\tWinfield\tWV\tPutnam County\tH1\n25560\t54079\tScott depot\tWV\tPutnam County\tH1\n25526\t54079\tHurricane\tWV\tPutnam County\tH1\n25510\t54079\tCulloden\tWV\tPutnam County\tH1\n25168\t54079\tRed house\tWV\tPutnam County\tH1\n25109\t54079\tHometown\tWV\tPutnam County\tH1\n25159\t54079\tPoca\tWV\tPutnam County\tH1\n25033\t54079\tBuffalo\tWV\tPutnam County\tH1\n25123\t54079\tLeon\tWV\tPutnam County\tH1\n25541\t54079\tMilton\tWV\tPutnam County\tH1\n25011\t54079\tBancroft\tWV\tPutnam County\tH1\n25177\t54079\tSaint albans\tWV\tPutnam County\tH1\n25082\t54079\tFraziers bottom\tWV\tPutnam County\tH1\n25245\t54079\tGiven\tWV\tPutnam County\tH1\n25248\t54079\tKenna\tWV\tPutnam County\tH1\n25124\t54079\tLiberty\tWV\tPutnam County\tH1\n25569\t54079\tTeays\tWV\tPutnam County\tH1\n25070\t54079\tEleanor\tWV\tPutnam County\tH1\n25140\t54081\tNaoma\tWV\tRaleigh County\tH1\n25918\t54081\tShady spring\tWV\tRaleigh County\tH1\n25825\t54081\tCool ridge\tWV\tRaleigh County\tH1\n25836\t54081\tEccles\tWV\tRaleigh County\tH1\n25209\t54081\tWhitesville\tWV\tRaleigh County\tH1\n25801\t54081\tBeckley\tWV\tRaleigh County\tH1\n25880\t54081\tMount hope\tWV\tRaleigh County\tH1\n25839\t54081\tFairdale\tWV\tRaleigh County\tH1\n25849\t54081\tGlen white\tWV\tRaleigh County\tH1\n25989\t54081\tWhite oak\tWV\tRaleigh County\tH1\n25909\t54081\tProsperity\tWV\tRaleigh County\tH1\n25932\t54081\tSurveyor\tWV\tRaleigh County\tH1\n25878\t54081\tMidway\tWV\tRaleigh County\tH1\n25827\t54081\tCrab orchard\tWV\tRaleigh County\tH1\n25813\t54081\tBeaver\tWV\tRaleigh County\tH1\n25951\t54081\tHinton\tWV\tRaleigh County\tH1\n25901\t54081\tOak hill\tWV\tRaleigh County\tH1\n25844\t54081\tGlen daniel\tWV\tRaleigh County\tH1\n25823\t54081\tCoal city\tWV\tRaleigh County\tH1\n25908\t54081\tPrincewick\tWV\tRaleigh County\tH1\n25860\t54081\tLanark\tWV\tRaleigh County\tH1\n25174\t54081\tRock creek\tWV\tRaleigh County\tH1\n25927\t54081\tStanaford\tWV\tRaleigh County\tH1\n25906\t54081\tPiney view\tWV\tRaleigh County\tH1\n25851\t54081\tHarper\tWV\tRaleigh County\tH1\n25007\t54081\tArnett\tWV\tRaleigh County\tH1\n25864\t54081\tLayland\tWV\tRaleigh County\tH1\n25865\t54081\tLester\tWV\tRaleigh County\tH1\n25969\t54081\tJumping branch\tWV\tRaleigh County\tH1\n25180\t54081\tSaxon\tWV\tRaleigh County\tH1\n25841\t54081\tFlat top\tWV\tRaleigh County\tH1\n25920\t54081\tSlab fork\tWV\tRaleigh County\tH1\n25919\t54081\tSkelton\tWV\tRaleigh County\tH1\n25871\t54081\tMabscott\tWV\tRaleigh County\tH1\n25843\t54081\tGhent\tWV\tRaleigh County\tH1\n25060\t54081\tDorothy\tWV\tRaleigh County\tH1\n25857\t54081\tJosephine\tWV\tRaleigh County\tH1\n25902\t54081\tOdd\tWV\tRaleigh County\tH1\n25817\t54081\tBolt\tWV\tRaleigh County\tH1\n25062\t54081\tDry creek\tWV\tRaleigh County\tH1\n25044\t54081\tClear creek\tWV\tRaleigh County\tH1\n25853\t54081\tHelen\tWV\tRaleigh County\tH1\n25832\t54081\tDaniels\tWV\tRaleigh County\tH1\n25915\t54081\tRhodell\tWV\tRaleigh County\tH1\n25911\t54081\tRaleigh\tWV\tRaleigh County\tH1\n25818\t54081\tBradley\tWV\tRaleigh County\tH1\n25873\t54081\tMac arthur\tWV\tRaleigh County\tH1\n25811\t54081\tAmigo\tWV\tRaleigh County\tH1\n25048\t54081\tColcord\tWV\tRaleigh County\tH1\n25802\t54081\tBeckley\tWV\tRaleigh County\tH1\n25008\t54081\tArtie\tWV\tRaleigh County\tH1\n25921\t54081\tSophia\tWV\tRaleigh County\tH1\n26267\t54083\tEllamore\tWV\tRandolph County\tH1\n26294\t54083\tValley head\tWV\tRandolph County\tH1\n26241\t54083\tElkins\tWV\tRandolph County\tH1\n26257\t54083\tCoalton\tWV\tRandolph County\tH1\n26253\t54083\tBeverly\tWV\tRandolph County\tH1\n26273\t54083\tHuttonsville\tWV\tRandolph County\tH1\n26296\t54083\tWhitmer\tWV\tRandolph County\tH1\n26268\t54083\tGlady\tWV\tRandolph County\tH1\n26263\t54083\tDryfork\tWV\tRandolph County\tH1\n26250\t54083\tBelington\tWV\tRandolph County\tH1\n26280\t54083\tMill creek\tWV\tRandolph County\tH1\n26254\t54083\tBowden\tWV\tRandolph County\tH1\n26285\t54083\tNorton\tWV\tRandolph County\tH1\n26230\t54083\tPickens\tWV\tRandolph County\tH1\n26283\t54083\tMontrose\tWV\tRandolph County\tH1\n26282\t54083\tMonterville\tWV\tRandolph County\tH1\n26293\t54083\tValley bend\tWV\tRandolph County\tH1\n26259\t54083\tDailey\tWV\tRandolph County\tH1\n26276\t54083\tKerens\tWV\tRandolph County\tH1\n26278\t54083\tMabie\tWV\tRandolph County\tH1\n26224\t54083\tHelvetia\tWV\tRandolph County\tH1\n26270\t54083\tHarman\tWV\tRandolph County\tH1\n26170\t54085\tSaint marys\tWV\tRitchie County\tH1\n26180\t54085\tWalker\tWV\tRitchie County\tH1\n26346\t54085\tEllenboro\tWV\tRitchie County\tH1\n26178\t54085\tSmithville\tWV\tRitchie County\tH1\n26415\t54085\tPennsboro\tWV\tRitchie County\tH1\n26456\t54085\tWest union\tWV\tRitchie County\tH1\n26362\t54085\tHarrisville\tWV\tRitchie County\tH1\n26421\t54085\tPullman\tWV\tRitchie County\tH1\n26137\t54085\tBig springs\tWV\tRitchie County\tH1\n26161\t54085\tPetroleum\tWV\tRitchie County\tH1\n26337\t54085\tCairo\tWV\tRitchie County\tH1\n26143\t54085\tElizabeth\tWV\tRitchie County\tH1\n26327\t54085\tBerea\tWV\tRitchie County\tH1\n26325\t54085\tAuburn\tWV\tRitchie County\tH1\n26148\t54085\tMacfarlan\tWV\tRitchie County\tH1\n26138\t54085\tBrohard\tWV\tRitchie County\tH1\n25071\t54087\tElkview\tWV\tRoane County\tH1\n25252\t54087\tLe roy\tWV\tRoane County\tH1\n25259\t54087\tLooneyville\tWV\tRoane County\tH1\n25005\t54087\tAmma\tWV\tRoane County\tH1\n25045\t54087\tClendenin\tWV\tRoane County\tH1\n25266\t54087\tNewton\tWV\tRoane County\tH1\n25286\t54087\tWalton\tWV\tRoane County\tH1\n25251\t54087\tLeft hand\tWV\tRoane County\tH1\n25164\t54087\tProcious\tWV\tRoane County\tH1\n25243\t54087\tGandeeville\tWV\tRoane County\tH1\n25276\t54087\tSpencer\tWV\tRoane County\tH1\n25270\t54087\tReedy\tWV\tRoane County\tH1\n24963\t54089\tPeterstown\tWV\tSummers County\tH1\n25918\t54089\tShady spring\tWV\tSummers County\tH1\n25825\t54089\tCool ridge\tWV\tSummers County\tH1\n25986\t54089\tSpring dale\tWV\tSummers County\tH1\n24918\t54089\tBallard\tWV\tSummers County\tH1\n25951\t54089\tHinton\tWV\tSummers County\tH1\n25977\t54089\tMeadow creek\tWV\tSummers County\tH1\n25969\t54089\tJumping branch\tWV\tSummers County\tH1\n25979\t54089\tPipestem\tWV\tSummers County\tH1\n24935\t54089\tForest hill\tWV\tSummers County\tH1\n24981\t54089\tTalcott\tWV\tSummers County\tH1\n25966\t54089\tGreen sulphur springs\tWV\tSummers County\tH1\n25978\t54089\tNimitz\tWV\tSummers County\tH1\n24985\t54089\tWayside\tWV\tSummers County\tH1\n25985\t54089\tSandstone\tWV\tSummers County\tH1\n25976\t54089\tMeadow bridge\tWV\tSummers County\tH1\n24910\t54089\tAlderson\tWV\tSummers County\tH1\n24962\t54089\t
